vi "begin stream read at least.vi"(5 "id":u32, 7 "event":refnum<user-event>, 8 "error in":errorcluster, 9 "max bytes to read":u32, 10 "min bytes to read":u32, 11 "socket":u64) -> (0 "error out":errorcluster)   [LabVIEW 2016, in "async tls.lvlib"]
uses:
  async tls.lvlib
  tls action complete user event.ctl
  lvasynctls.dll
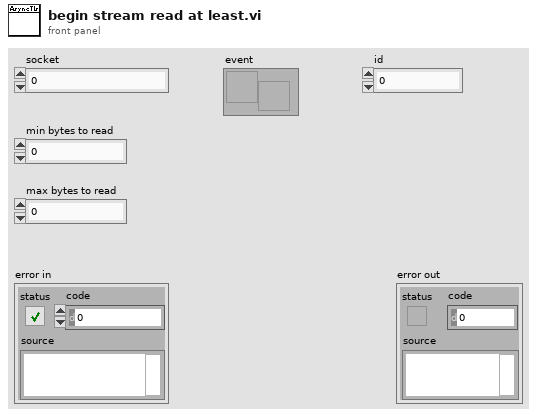
[diagram p1: front panel]
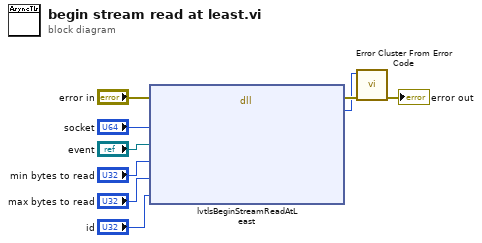
[diagram p0: block diagram]
diagram:
  n1 = dll-call lib="C:/Users/IEUser/Desktop/libasynclvtls/lvasynctls.dll" fn="lvtlsBeginStreamReadAtLeast"(error in="error in", "socket"="socket", "event"="event", "min bytes to read"="min bytes to read", "max bytes to read"="max bytes to read", "id"="id") -> (error out=w9:errorcluster, "err"=w8:i32)  [unwired: 7 in, 1 out]
  n2 = call <vilib>:"Error Cluster From Error Code.vi"("error in (no error)"=w9, "error code (0)"=w8) -> ("error out"=→"error out":errorcluster)  [unwired: 7 in]
